vi "RotationApplication v6.vi"() -> ()   [LabVIEW 2012]
uses:
  <instrlib>/ZaberTSeries/Public/Utility/Request.ctl
  <instrlib>/ZaberTSeries/Public/Utility/Response.ctl
  variables/GlobalUI.vi
  <vilib>/Utility/file.llb/Write To Spreadsheet File (string).vi
  Stage Global.vi
  <instrlib>/ZaberTSeries/ZaberTSeries.lvlib
panel:
  in  "OriginalFormula":string
  in  "Restore":bool
  in  "Calibrate":bool
  out "Scanning?":bool
  out "Current Angle (deg)":dbl=45.0
  out "Stage Position (mm)":dbl=76.5
  in  "Time Step (ms)":dbl
  in  "Rotation f(x) (mm -> deg)":string="1*x + -1080.000000"
  in  "Finish Rotation f(x)":bool
  in  "Scan":bool
  in  "stop":bool
  in  "Go Home":bool
  in  "Set Home Offset":dbl=80.0
  in  "TabControl":T1(tab)
  in  "Optimize":bool
  in  "Angle?":bool
  out "Current Angle (deg)":dbl=52.314375
  in  "Move Rel?":bool
  in  "Move Abs?":bool
  in  "Move Rel (deg)":dbl=-1.0 step=0.1
  in  "Move Abs (deg)":dbl=35.0
  in  "Send":bool
  out "Command?":bool=TRUE
  in  "REQUEST:":T2={"Device Number"=1, "Command"=23, "Data"=-10000, "Response Count"=1} {"Command" items=["Echo"=55, "Home"=1, "Move Absolute"=20, "Move Relative"=21, "Move at Constant Speed"=22, "Renumber"=2, "Restore Settings"=36, "Stop"=23]}
  out "Response Data:":T3 {"Command" items=["Constant Speed Tracking"=8, "Echo"=55, "Error"=255, "Home"=1, "Limit Active"=9, "Manual Move Tracking"=10, "Move Absolute"=20, "Move at Constant Speed"=22, "Move Relative"=21, "Renumber"=2, "Restore Settings"=36, "Stop"=23]}
  in  "Command":bool
  in  "DONE":bool
  in  "angle":dbl=7.89375
  in  "Aquire AngleScan":bool
  out "Intensity vs Angle Plot":cluster{dbl[], dbl[]}(graph)={[0.1003125, 0.200625, 0.30093749999999997, 0.40125, 0.5015625, 0.6018749999999999, 0.7021875, 0.8025, 0.9028125, 1.003125, 1.1034374999999998, 1.2037499999999999, 1.3040625, 1.404375, 1.5046875, 1.605, 1.7053125, 1.805625, 1.9059374999999998, 2.00625, 2.1065625, 2.2068749999999997, 2.3071875, 2.4074999999999998, 2.5078125, 2.608125, 2.7084375, 2.80875, 2.9090625, 3.009375, 3.1096874999999997, 3.21, 3.3103124999999998, 3.410625, 3.5109375, 3.61125, 3.7115625, 3.8118749999999997, 3.9121875, 4.0125, 4.1128124999999995, 4.213125, 4.3134375, 4.413749999999999], [0.10330483041158461, 0.10354301638719464, 0.10354301638719464, 0.10358827172256029, 0.10358827172256029, 0.10288562309451152, 0.10288562309451152, 0.10288562309451152, 0.1017709127286577, 0.1017709127286577, 0.10044183498475528, 0.09877691501524301, 0.09877691501524301, 0.10001548208841382, 0.10001548208841382, 0.09941763528963352, 0.09941763528963352, 0.09897222751524294, 0.09965820312499914, 0.09965820312499914, 0.09993807164634047, 0.09985708841463325, 0.09985708841463325, 0.09985708841463325, 0.10042158917682856, 0.10075624047256009, 0.10075624047256009, 0.10102419969512122, 0.1007193216463409, 0.1007193216463409, 0.1007193216463409, 0.10111828315548696, 0.10111828315548696, 0.10111828315548696, 0.10066811166158449, 0.10066811166158449, 0.10040610708841394, 0.10110399199695043, 0.10110399199695043, 0.10115996570121859, 0.10115996570121859, 0.10151248094512112, 0.10151248094512112, 0.10125047637195043]}
  in  "Step Size (deg)":dbl=1.0
  in  "Final Angle (deg)":dbl=45.0
  in  "Initial Angle (deg)":dbl
  in  "Activate AngleScan":bool
  out "Calibrate?":bool
  in  "ABORT":bool
  out "File Destination":path
  in  "Initialize AngleScan":bool
  in  "Simulation":bool
  out "Simulate?":bool
  in  "Finish Stage":bool
  in  "Start/pause":bool
  in  "Start/Pause Stage":bool
  out "Current Position (mm)":dbl
  in  "Finish Rotation":bool
  out "Current Angle":dbl
  in  "Initial Position (mm)":dbl
  in  "Final Position (mm)":dbl
  in  "Number of Steps":u32
  in  "Speed (um/s)":dbl
  in  "Final Angle (deg)":dbl=45.0
  in  "Number of Rotations":u32=4500
  in  "Polynomial Degree":dbl=1.0
  in  "VISA reference name:":refnum<visa-resource-name>="COM4"
  # "==>"
  # "Device"
  # "Command (Binary)"
  # "Data"
  # "==>"
  # "Data"
  # "==>"
  # "Rotation Mount Settings:"
  # "Simulated Delay Stage Settings:"
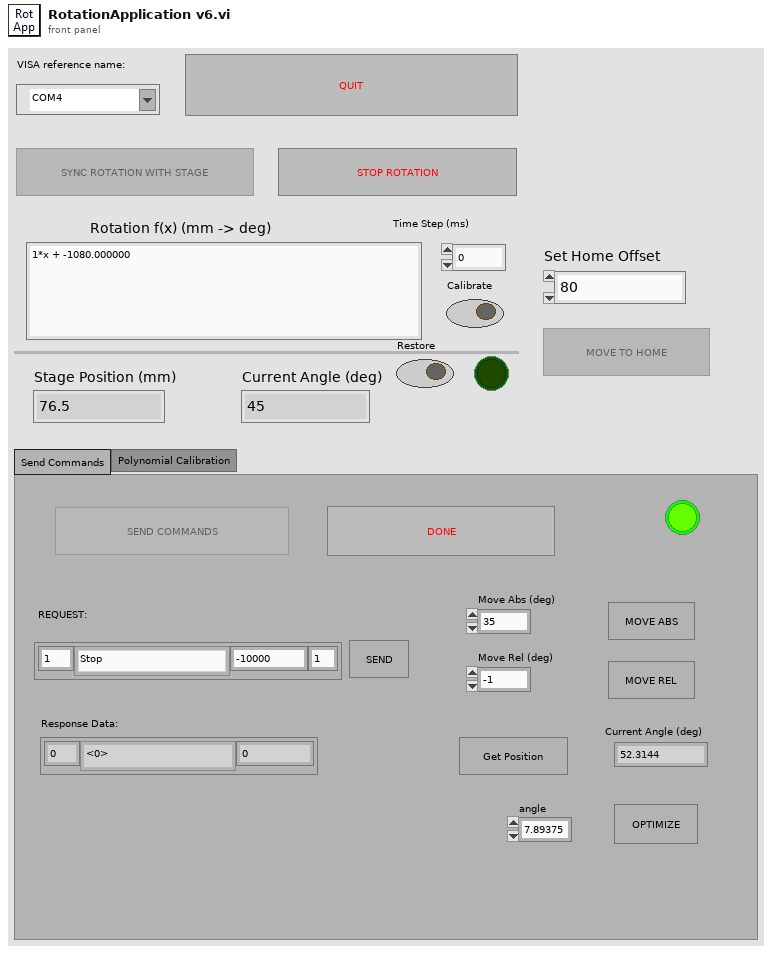
[diagram p1: front panel]
types:
  T1 = enum32{"Send Commands", "Polynomial Calibration", "Simulated f(x)  ", "Adjust Simulation Settings"}
  T2 = typedef "ZaberTSeries.lvlib/Request.ctl" = cluster{"Device Number":u8, "Command":u8, "Data":i32, "Response Count":i32}
  T3 = typedef "ZaberTSeries.lvlib/Response.ctl" = cluster{"Device Number":u8, "Command":u8, "Data":i32}
  T4 = enum8{"Enabled", "Disabled", "Disabled and Grayed Out"}
  T5 = typedef "Scan Parameters.ctl" = cluster{"x pixels":i32, "x voltage min":dbl, "x voltage max":dbl, "y voltage min":dbl, "y voltage max":dbl, "fill frac":dbl, "Zoom":dbl, "BiDi":bool, "scan rate (ms/line)":dbl}
  T6 = typedef "Stage Parameters.ctl" = cluster{"Scan Mode":T7, "Start position mm":dbl, "End position mm":dbl, "Velocity um/sec (continuous)":dbl, "Step size microns (discrete)":dbl, "Frames to grab (grab)":i32, "Sync Rotation with Stage":bool}
  T7 = typedef "ScanMode.ctl" = enum16{"None", "Continuous", "Point Scan (CH3 cursor)", "Point Scan Move (CH3 cursor)", "Grab", "Grab Move Stage", "Grab Move Z-stage", "Cont. Move Z-stage", "Spec Move Stage", "Spec Move Cont", "Surf Calib"}
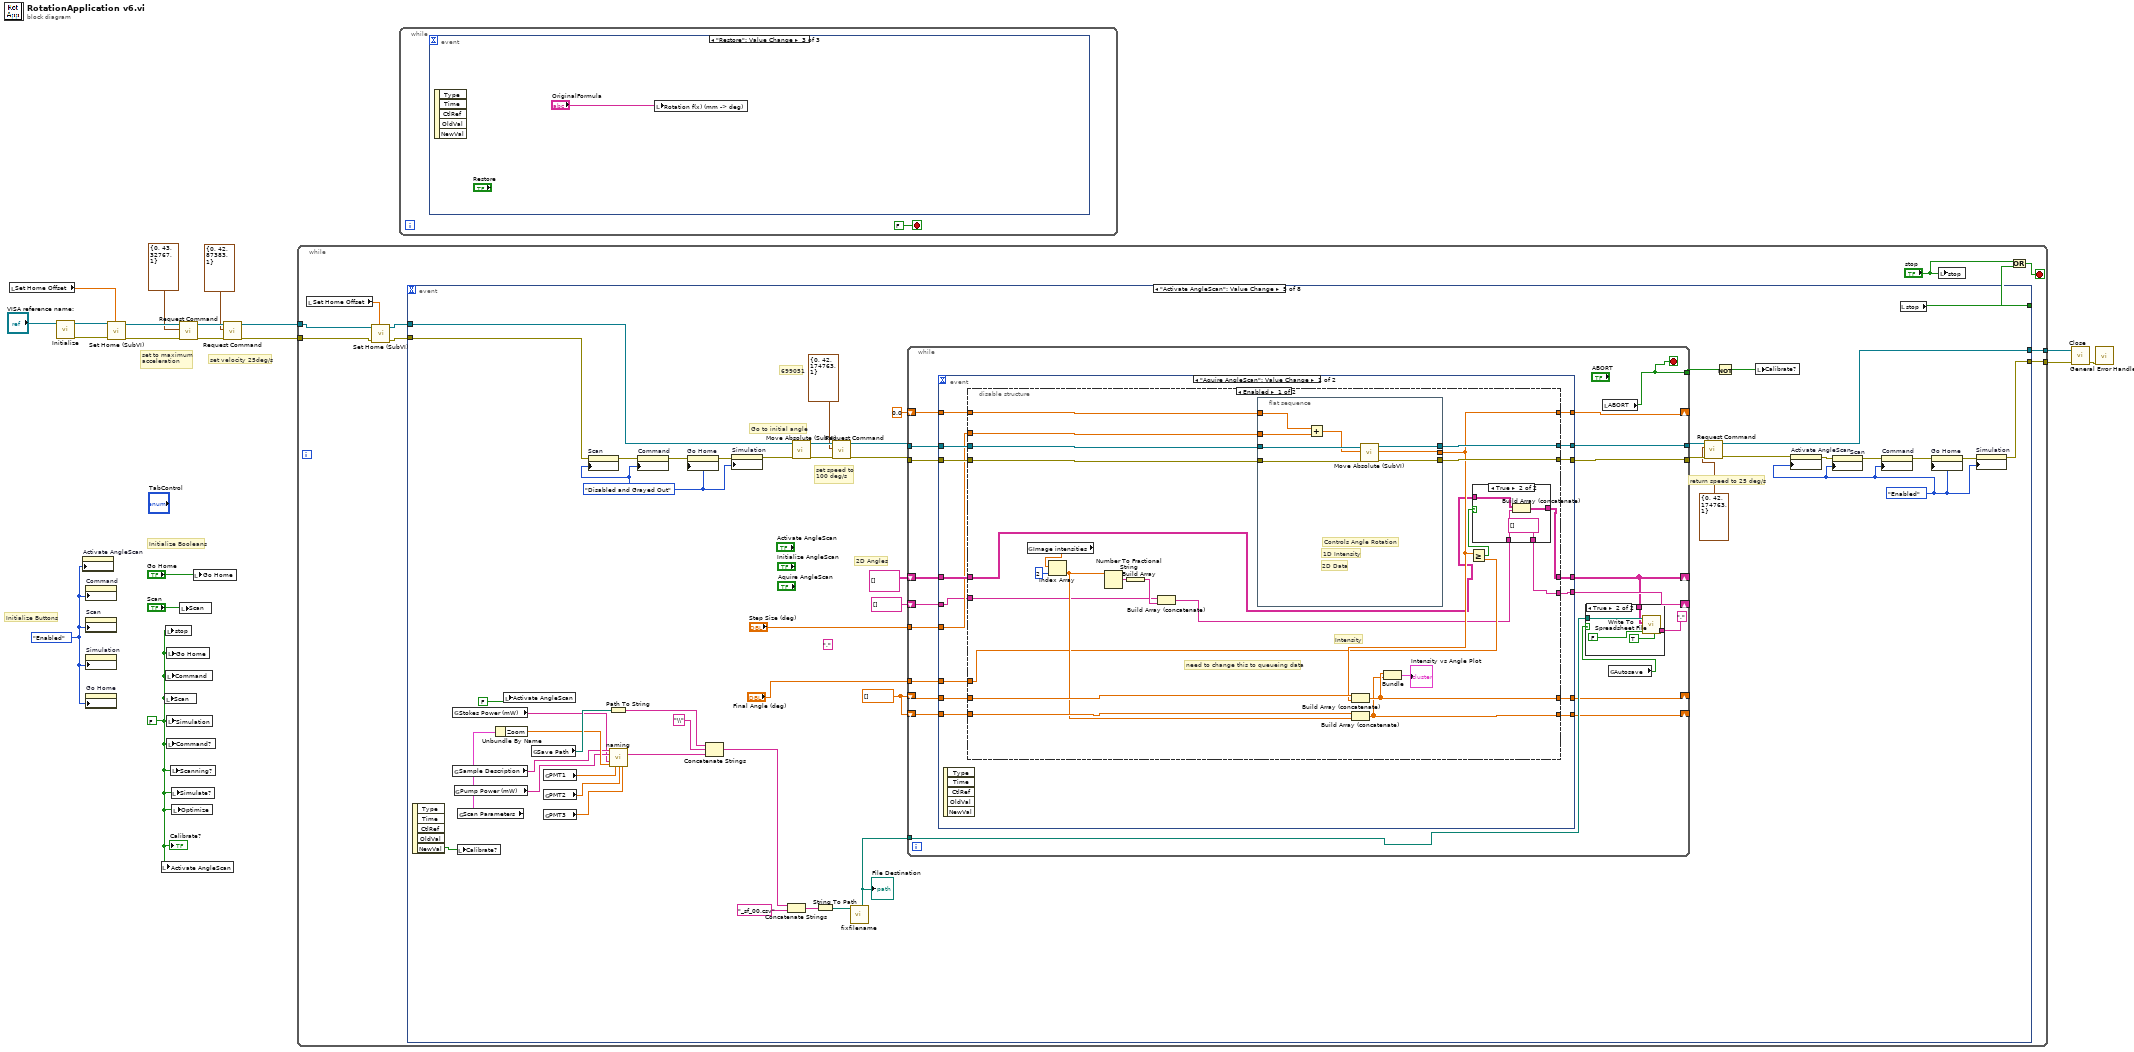
[diagram p0: block diagram]
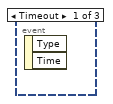
[diagram p2: hidden frame]
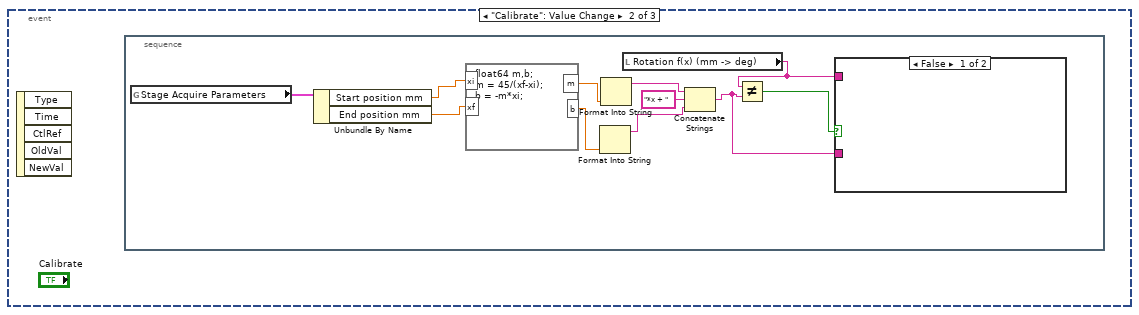
[diagram p3: hidden frame]
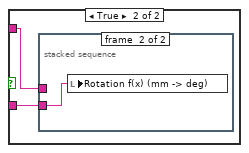
[diagram p4: hidden frame]
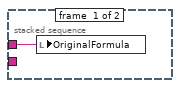
[diagram p5: hidden frame]
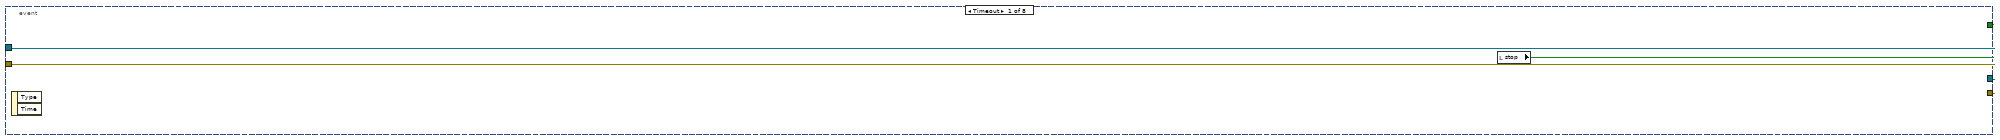
[diagram p6: hidden frame]
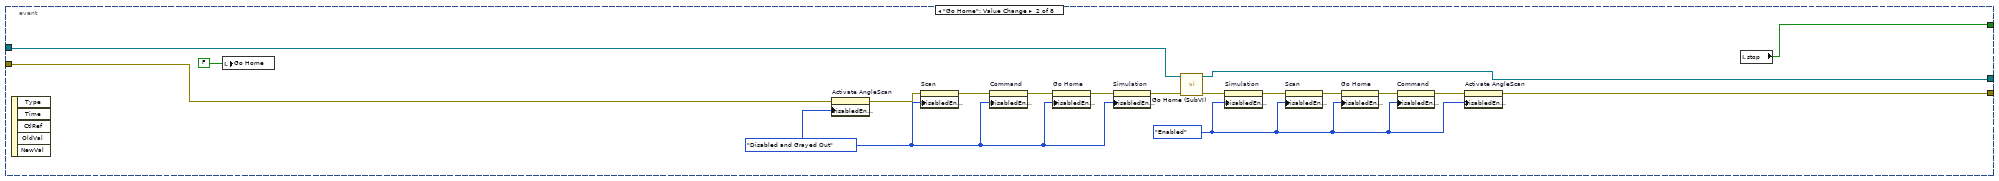
[diagram p7: hidden frame]
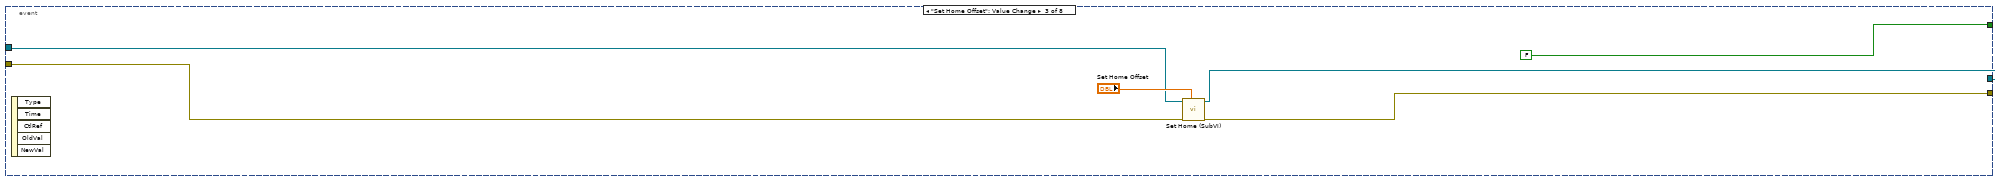
[diagram p8: hidden frame]
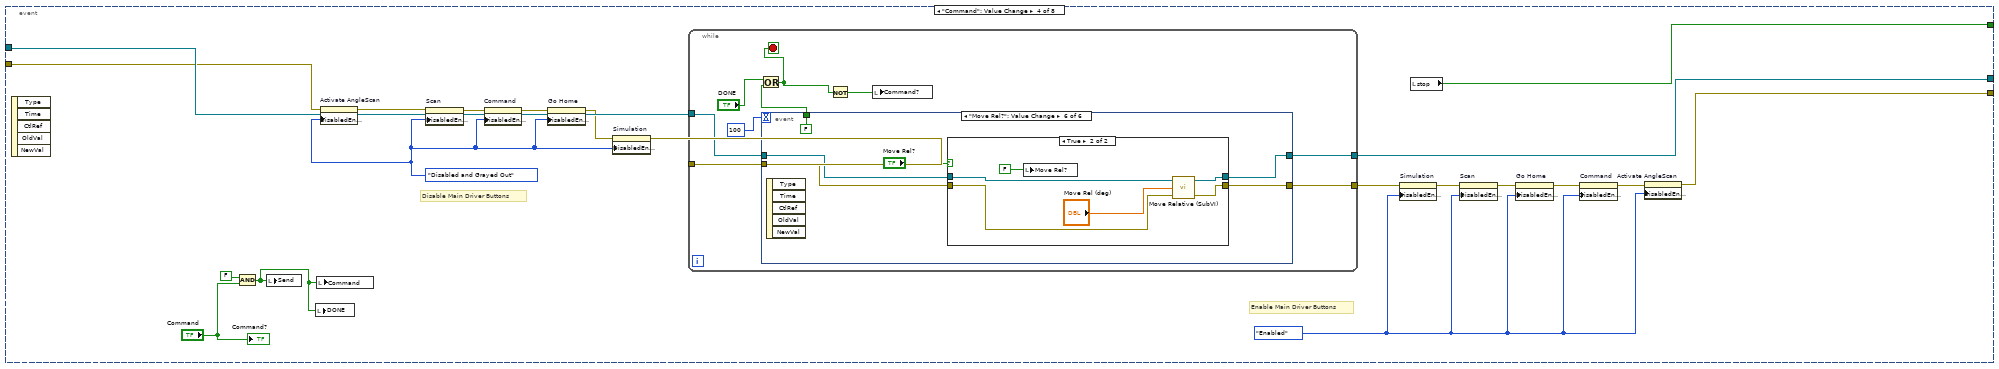
[diagram p9: hidden frame]
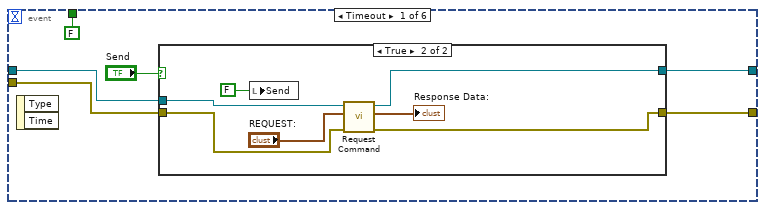
[diagram p10: hidden frame]
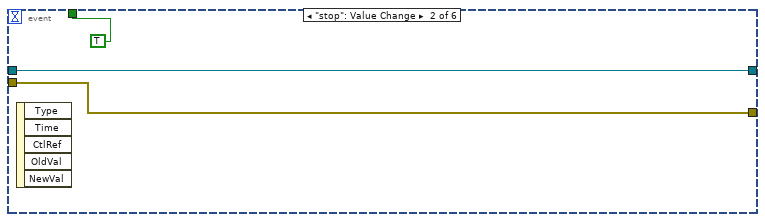
[diagram p12: hidden frame]
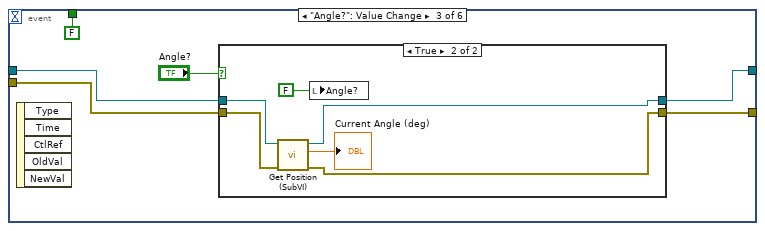
[diagram p13: hidden frame]
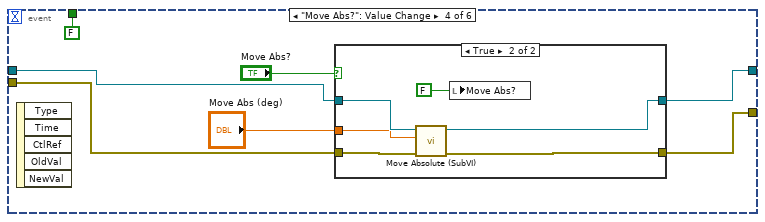
[diagram p15: hidden frame]
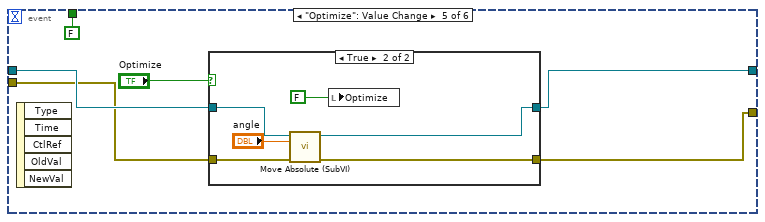
[diagram p17: hidden frame]
diagram:
  w9 = T4."Enabled" ("Disabled")
  w10 = FALSE ("y")
  # "set to maximum\nacceleration"
  # "set velocity 25deg/s"
  # "Initialize Buttons"
  # "Initialize Booleans"
  n1 = local read "Set Home Offset"() -> (w11:dbl)
  n2 = call <instrlib>:"Initialize.vi"("VISA resource name"="VISA reference name:") -> ("error out"=w12:errorcluster, "VISA resource name out"=w13:refnum<visa-resource-name>)  [unwired: 8 in, 1 out]
  n3 = property on="Activate AngleScan" class="Bool (strict)"("DisabledEnum"=w9) -> ()  [unwired: 2 in, 2 out]
  n4 = property on="Command" class="Bool (strict)"("DisabledEnum"=w9) -> ()  [unwired: 2 in, 2 out]
  n5 = property on="Scan" class="Bool (strict)"("DisabledEnum"=w9) -> ()  [unwired: 2 in, 2 out]
  n6 = property on="Simulation" class="Bool (strict)"("DisabledEnum"=w9) -> ()  [unwired: 2 in, 2 out]
  n7 = property on="Go Home" class="Bool (strict)"("DisabledEnum"=w9) -> ()  [unwired: 2 in, 2 out]
  n8 = call "Set Home (SubVI).vi"("Home Offset (deg)"=w11, "error in (no error)"=w12, "VISA Refnum in"=w13) -> ("error out"=w7:errorcluster, "VISA Refnum out"=w8:refnum<visa-resource-name>)  [unwired: 7 in]
  n9 = local write "Activate AngleScan"(w10) -> ()
  n10 = local write "Scan"(w10) -> ()
  n11 = local write "stop"(w10) -> ()
  n12 = local write "Command"(w10) -> ()
  n13 = local write "Go Home"(w10) -> ()
  n14 = local write "Simulation"(w10) -> ()
  n15 = local write "Command?"(w10) -> ()
  n16 = local write "Scanning?"(w10) -> ()
  n17 = local write "Simulate?"(w10) -> ()
  n18 = local write "Optimize"(w10) -> ()
  n19 = call <instrlib>:"Request Command.vi"("error in (no error)"=w7, "Request"=T2 {"Device Number"=0, "Command"=43, "Data"=32767, "Response Count"=1}, "VISA resource name"=w8) -> ("error out"=w5:errorcluster, "VISA resource name out"=w6:refnum<visa-resource-name>)  [unwired: 5 in, 2 out]
  n20 = local write "Scan"("Scan") -> ()
  n21 = local write "Go Home"("Go Home") -> ()
  n22 = call <instrlib>:"Request Command.vi"("error in (no error)"=w5, "Request"=T2 {"Device Number"=0, "Command"=42, "Data"=87383, "Response Count"=1}, "VISA resource name"=w6) -> ("error out"=w3:errorcluster, "VISA resource name out"=w4:refnum<visa-resource-name>)  [unwired: 5 in, 2 out]
  n23 = while {
    tunnel: w4 -> [w23]
    tunnel: w3 -> [w20]
    tunnel: [w29] -> w17
    tunnel: [w28] -> w19
    stop <- w27 stop-if-true
    n24 = local read "Set Home Offset"() -> (w24:dbl)
    n25 = call "Set Home (SubVI).vi"("Home Offset (deg)"=w24, "error in (no error)"=w20, "VISA Refnum in"=w23) -> ("error out"=w21:errorcluster, "VISA Refnum out"=w22:refnum<visa-resource-name>)  [unwired: 7 in]
    n26 = event shown="[4] \"Activate AngleScan\": Value Change" {
      selector: _ -> [_ _ _ _ _ _ _ _]
      dyn-events: _ -> [_ _ _ _ _ _ _ _]
      timeout: _ -> [_ _ _ _ _ _ _ _]
      tunnel: w22 -> [w32 w45 w55 w76 w201 w389 w419 w486]
      tunnel: w21 -> [w31 w36 w54 w62 w205 w386 w404 w485]
      tunnel: [w32 w40 w53 w68 w169 w388 w426 w486] -> w28
      tunnel: [w31 w33 w52 w57 w189 w370 w423 w485] -> w29
      tunnel: [w30 w50 FALSE ("stop") w75 w211 w390 w430 w487] -> w26
      event Timeout {
        n27 = event-data() -> ()  [unwired: 1 in, 2 out]
        n28 = local read "stop"() -> (w30:bool)
      }
      event "Go Home": Value Change {
        w34 = T4."Enabled" ("Disabled")
        w38 = T4."Disabled and Grayed Out" ("Disabled")
        n29 = event-data() -> ()  [unwired: 1 in, 5 out]
        n30 = local write "Go Home"(FALSE ("Go Home")) -> ()
        n31 = property on="Activate AngleScan" class="Bool (strict)"(error in=w36, "DisabledEnum"=w38) -> (error out=w37:errorcluster)  [unwired: 1 in, 1 out]
        n32 = property on="Scan" class="Bool (strict)"(error in=w37, "DisabledEnum"=w38) -> (error out=w48:errorcluster)  [unwired: 1 in, 1 out]
        n33 = property on="Command" class="Bool (strict)"(error in=w48, "DisabledEnum"=w38) -> (error out=w47:errorcluster)  [unwired: 1 in, 1 out]
        n34 = property on="Go Home" class="Bool (strict)"(error in=w47, "DisabledEnum"=w38) -> (error out=w46:errorcluster)  [unwired: 1 in, 1 out]
        n35 = property on="Simulation" class="Bool (strict)"(error in=w46, "DisabledEnum"=w38) -> (error out=w44:errorcluster)  [unwired: 1 in, 1 out]
        n36 = call "Go Home (SubVI).vi"("error in (no error)"=w44, "VISA Refnum in"=w45) -> ("error out"=w39:errorcluster, "VISA Refnum out"=w40:refnum<visa-resource-name>)  [unwired: 8 in]
        n37 = property on="Simulation" class="Bool (strict)"(error in=w39, "DisabledEnum"=w34) -> (error out=w41:errorcluster)  [unwired: 1 in, 1 out]
        n38 = property on="Scan" class="Bool (strict)"(error in=w41, "DisabledEnum"=w34) -> (error out=w43:errorcluster)  [unwired: 1 in, 1 out]
        n39 = property on="Go Home" class="Bool (strict)"(error in=w43, "DisabledEnum"=w34) -> (error out=w42:errorcluster)  [unwired: 1 in, 1 out]
        n40 = property on="Command" class="Bool (strict)"(error in=w42, "DisabledEnum"=w34) -> (error out=w35:errorcluster)  [unwired: 1 in, 1 out]
        n41 = property on="Activate AngleScan" class="Bool (strict)"(error in=w35, "DisabledEnum"=w34) -> (error out=w33:errorcluster)  [unwired: 1 in, 1 out]
        n42 = local read "stop"() -> (w50:bool)
      }
      event "Set Home Offset": Value Change {
        n43 = event-data() -> ()  [unwired: 1 in, 5 out]
        n44 = call "Set Home (SubVI).vi"("Home Offset (deg)"="Set Home Offset", "error in (no error)"=w54, "VISA Refnum in"=w55) -> ("error out"=w52:errorcluster, "VISA Refnum out"=w53:refnum<visa-resource-name>)  [unwired: 7 in]
      }
      event "Command": Value Change {
        w59 = T4."Enabled" ("Disabled")
        w60 = T4."Disabled and Grayed Out" ("Disabled")
        # "Enable Main Driver Buttons"
        # "Disable Main Driver Buttons"
        n45 = event-data() -> ()  [unwired: 1 in, 5 out]
        n46 = And(x=FALSE ("Command"), y="Command") -> (x .and. y?=w64:bool)
        n47 = local write "Send"(w64) -> ()
        n48 = local write "DONE"(w64) -> ()
        n49 = local write "Command"(w64) -> ()
        n50 = property on="Activate AngleScan" class="Bool (strict)"(error in=w62, "DisabledEnum"=w60) -> (error out=w61:errorcluster)  [unwired: 1 in, 1 out]
        n51 = property on="Scan" class="Bool (strict)"(error in=w61, "DisabledEnum"=w60) -> (error out=w70:errorcluster)  [unwired: 1 in, 1 out]
        n52 = property on="Command" class="Bool (strict)"(error in=w70, "DisabledEnum"=w60) -> (error out=w71:errorcluster)  [unwired: 1 in, 1 out]
        n53 = property on="Go Home" class="Bool (strict)"(error in=w71, "DisabledEnum"=w60) -> (error out=w72:errorcluster)  [unwired: 1 in, 1 out]
        n54 = property on="Simulation" class="Bool (strict)"(error in=w72, "DisabledEnum"=w60) -> (error out=w69:errorcluster)  [unwired: 1 in, 1 out]
        n55 = while {
          tunnel: w76 -> [w82]
          tunnel: [w85] -> w68
          tunnel: w69 -> [w81]
          tunnel: [w84] -> w63
          stop <- w78 stop-if-true
          n56 = event shown="[5] \"Move Rel?\": Value Change" {
            selector: _ -> [_ _ _ _ _ _]
            dyn-events: _ -> [_ _ _ _ _ _]
            timeout: 100 -> [_ _ _ _ _ _]
            tunnel: [w91 w102 w108 w121 w135 w149] -> w85
            tunnel: [w90 w103 w105 w119 w134 w148] -> w84
            tunnel: w82 -> [w88 w102 w107 w122 w137 w151]
            tunnel: w81 -> [w87 w103 w106 w120 w136 w150]
            tunnel: [FALSE TRUE FALSE FALSE FALSE FALSE] -> w77
            event Timeout {
              n57 = event-data() -> ()  [unwired: 1 in, 2 out]
              n58 = case shown="True" "Send" {
                tunnel: w88 -> [w93 w99]
                tunnel: [w93 w98] -> w91
                tunnel: w87 -> [w92 w97]
                tunnel: [w92 w96] -> w90
                frame False {
                }
                frame True {
                  n59 = local write "Send"(FALSE ("Send")) -> ()
                  n60 = call <instrlib>:"Request Command.vi"("error in (no error)"=w97, "Request"="REQUEST:", "VISA resource name"=w99) -> ("error out"=w96:errorcluster, "First Response"=→"Response Data:":T3, "VISA resource name out"=w98:refnum<visa-resource-name>)  [unwired: 5 in, 1 out]
                }
              }
            }
            event "stop": Value Change {
              n61 = event-data() -> ()  [unwired: 1 in, 5 out]
            }
            event "Angle?": Value Change {
              n62 = event-data() -> ()  [unwired: 1 in, 5 out]
              n63 = case shown="True" "Angle?" {
                tunnel: [w111 w116] -> w108
                tunnel: w107 -> [w111 w115]
                tunnel: w106 -> [w110 w114]
                tunnel: [w110 w113] -> w105
                frame False {
                }
                frame True {
                  n64 = call "Get Position (SubVI).vi"("error in (no error)"=w114, "VISA Refnum in"=w115) -> ("error out"=w113:errorcluster, "Position"=→"Current Angle (deg)":dbl, "VISA Refnum out"=w116:refnum<visa-resource-name>)  [unwired: 7 in]
                  n65 = local write "Angle?"(FALSE ("Angle?")) -> ()
                }
              }
            }
            event "Move Abs?": Value Change {
              n66 = event-data() -> ()  [unwired: 1 in, 5 out]
              n67 = case shown="True" "Move Abs?" {
                tunnel: "Move Abs (deg)" -> [_ w128]
                tunnel: w122 -> [w126 w132]
                tunnel: [w126 w131] -> w121
                tunnel: w120 -> [w125 w130]
                tunnel: [w125 w129] -> w119
                frame False {
                }
                frame True {
                  n68 = call "Move Absolute (SubVI).vi"("error in (no error)"=w130, "Move to Angle"=w128, "VISA Refnum in"=w132) -> ("error out"=w129:errorcluster, "VISA Refnum out"=w131:refnum<visa-resource-name>)  [unwired: 6 in, 1 out]
                  n69 = local write "Move Abs?"(FALSE ("Move Abs?")) -> ()
                }
              }
            }
            event "Optimize": Value Change {
              n70 = event-data() -> ()  [unwired: 1 in, 5 out]
              n71 = case shown="True" "Optimize" {
                tunnel: w137 -> [w140 w146]
                tunnel: [w140 w145] -> w135
                tunnel: w136 -> [w139 w144]
                tunnel: [w139 w143] -> w134
                frame False {
                }
                frame True {
                  n72 = call "Move Absolute (SubVI).vi"("error in (no error)"=w144, "Move to Angle"="angle", "VISA Refnum in"=w146) -> ("error out"=w143:errorcluster, "VISA Refnum out"=w145:refnum<visa-resource-name>)  [unwired: 6 in, 1 out]
                  n73 = local write "Optimize"(FALSE ("Move Abs?")) -> ()
                }
              }
            }
            event "Move Rel?": Value Change {
              n74 = event-data() -> ()  [unwired: 1 in, 5 out]
              n75 = case shown="True" "Move Rel?" {
                tunnel: w151 -> [w154 w159]
                tunnel: w150 -> [w153 w158]
                tunnel: [w154 w156] -> w149
                tunnel: [w153 w157] -> w148
                frame False {
                }
                frame True {
                  n76 = local write "Move Rel?"(FALSE ("Move Rel?")) -> ()
                  n77 = call "Move Relative (SubVI).vi"("error in (no error)"=w158, "Degrees to move"="Move Rel (deg)", "VISA resource name"=w159) -> ("error out"=w157:errorcluster, "VISA resource name out"=w156:refnum<visa-resource-name>)  [unwired: 1 out]
                }
              }
            }
          }
          n78 = Or(x="DONE", y=w77) -> (x .or. y?=w78:bool)
          n79 = Not(x=w78) -> (.not. x?=w83:bool)
          n80 = local write "Command?"(w83) -> ()
        }
        n81 = property on="Simulation" class="Bool (strict)"(error in=w63, "DisabledEnum"=w59) -> (error out=w65:errorcluster)  [unwired: 1 in, 1 out]
        n82 = local read "stop"() -> (w75:bool)
        n83 = property on="Scan" class="Bool (strict)"(error in=w65, "DisabledEnum"=w59) -> (error out=w67:errorcluster)  [unwired: 1 in, 1 out]
        n84 = property on="Go Home" class="Bool (strict)"(error in=w67, "DisabledEnum"=w59) -> (error out=w66:errorcluster)  [unwired: 1 in, 1 out]
        n85 = property on="Command" class="Bool (strict)"(error in=w66, "DisabledEnum"=w59) -> (error out=w58:errorcluster)  [unwired: 1 in, 1 out]
        n86 = property on="Activate AngleScan" class="Bool (strict)"(error in=w58, "DisabledEnum"=w59) -> (error out=w57:errorcluster)  [unwired: 1 in, 1 out]
        "Command?" <- "Command"
      }
      event "Activate AngleScan": Value Change {
        w171 = dbl[] []
        (unwired) "," ("delimiter (\\t)")
        w198 = T4."Enabled" ("Disabled")
        w199 = T4."Disabled and Grayed Out" ("Disabled")
        # "return speed to 25 deg/s"
        # "699051"
        # "set speed to\n100 deg/s"
        # "2D Angles"
        # "Go to initial angle"
        n87 = event-data() -> ("NewVal"=w210:bool)  [unwired: 1 in, 4 out]
        n88 = global read "GlobalUI.vi" "Stokes Power (mW)"() -> (w174:string)
        n89 = global read "GlobalUI.vi" "Sample Description"() -> (w176:string)
        n90 = global read "GlobalUI.vi" "Pump Power (mW)"() -> (w175:string)
        n91 = local write "Calibrate?"(w210) -> ()
        n92 = global read "GlobalUI.vi" "Scan Parameters"() -> (w178:T5)
        n93 = Unbundle By Name(w178) -> ("Zoom"=w177:dbl)
        n94 = local write "Activate AngleScan"(FALSE ("Scan Angles")) -> ()
        n95 = global read "GlobalUI.vi" "Save Path"() -> (w182:path)
        n96 = global read "GlobalUI.vi" "PMT1"() -> (w181:dbl)
        n97 = global read "GlobalUI.vi" "PMT2"() -> (w180:dbl)
        n98 = global read "GlobalUI.vi" "PMT3"() -> (w179:dbl)
        n99 = property on="Scan" class="Bool (strict)"(error in=w205, "DisabledEnum"=w199) -> (error out=w207:errorcluster)  [unwired: 1 in, 1 out]
        n100 = Path To String(path=w182) -> (string=w187:string)
        n101 = call "naming.vi"("Sample Description"=w176, "Pump Power (mW)"=w175, "Stokes Power (mW)"=w174, "Zoom"=w177, "PMT1"=w181, "PMT2"=w180, "PMT3"=w179) -> ("filename"=w173:string)  [unwired: 8 in]
        n102 = property on="Command" class="Bool (strict)"(error in=w207, "DisabledEnum"=w199) -> (error out=w208:errorcluster)  [unwired: 1 in, 1 out]
        n103 = property on="Go Home" class="Bool (strict)"(error in=w208, "DisabledEnum"=w199) -> (error out=w206:errorcluster)  [unwired: 1 in, 1 out]
        n104 = Concatenate Strings(w187, "\\" ("string"), w173) -> (w183:string)
        n105 = property on="Simulation" class="Bool (strict)"(error in=w206, "DisabledEnum"=w199) -> (error out=w200:errorcluster)  [unwired: 1 in, 1 out]
        n106 = Concatenate Strings(w183, "_sf_00.csv" ("string")) -> (w185:string)
        n107 = call "Move Absolute (SubVI).vi"("error in (no error)"=w200, "VISA Refnum in"=w201) -> ("error out"=w191:errorcluster, "VISA Refnum out"=w194:refnum<visa-resource-name>)  [unwired: 7 in, 1 out]
        n108 = String To Path(string=w185) -> (path=w184:path)
        n109 = call <instrlib>:"Request Command.vi"("error in (no error)"=w191, "Request"=T2 {"Device Number"=0, "Command"=42, "Data"=174763, "Response Count"=1}, "VISA resource name"=w194) -> ("error out"=w192:errorcluster, "VISA resource name out"=w193:refnum<visa-resource-name>)  [unwired: 5 in, 2 out]
        n110 = call "fixfilename.vi"("Path"=w184) -> ("fixed path"=w172:path)  [unwired: 9 in, 1 out]
        "File Destination" <- w172
        n111 = while {
          tunnel: "Final Angle (deg)" -> [w230]
          tunnel: w192 -> [w231]
          tunnel: [w217] -> w168
          tunnel: [w218] -> w170
          shift-right: [w213] -> _
          shift-left: string[][] [] -> [w229]
          tunnel: [w225] -> w197
          tunnel: w193 -> [w228]
          tunnel: w172 -> [w226]
          shift-right: [w224] -> _
          shift-left: 0.0 ("Initial Angle (deg)") -> [w223]
          shift-right: [w220] -> _
          shift-left: w171 -> [w222]
          shift-right: [w219] -> _
          shift-left: w171 -> [w221]
          tunnel: "Step Size (deg)" -> [w216]
          shift-right: [w215] -> _
          shift-left: string[] [] -> [w214]
          stop <- w225 stop-if-true
          n112 = event shown="[0] \"Aquire AngleScan\": Value Change" {
            selector: _ -> [_ _]
            dyn-events: _ -> [_ _]
            timeout: _ -> [_ _]
            tunnel: w228 -> [w252 _]
            tunnel: w231 -> [w251 _]
            tunnel: [w250 _] -> w218
            tunnel: [w249 _] -> w217
            tunnel: w230 -> [w248 w358]
            tunnel: w223 -> [w246 _]
            tunnel: w229 -> [w247 _]
            tunnel: [w245 w350] -> w213
            tunnel: [w244 "Initial Angle (deg)"] -> w224
            tunnel: w222 -> [w243 _]
            tunnel: w221 -> [w242 _]
            tunnel: [w241 _] -> w220
            tunnel: [w240 _] -> w219
            tunnel: w216 -> [w239 w354]
            tunnel: [w237 w351] -> w215
            tunnel: w214 -> [w238 _]
            event "Aquire AngleScan": Value Change {
              n113 = event-data() -> ()  [unwired: 1 in, 5 out]
              n114 = disable-structure shown="Enabled" {
                disable-tunnel: w239 -> [w261 w313]
                disable-tunnel: w252 -> [w276 w312]
                disable-tunnel: w251 -> [w275 w311]
                disable-tunnel: [w274 w310] -> w250
                disable-tunnel: [w273 w309] -> w249
                disable-tunnel: w248 -> [w258 w308]
                disable-tunnel: w247 -> [w256 w307]
                disable-tunnel: w246 -> [w272 w298]
                disable-tunnel: [w254 w296] -> w245
                disable-tunnel: [w259 w294] -> w244
                disable-tunnel: w243 -> [w271 _]
                disable-tunnel: w242 -> [w270 _]
                disable-tunnel: [w269 w293] -> w241
                disable-tunnel: [w268 w292] -> w240
                disable-tunnel: w238 -> [w260 _]
                disable-tunnel: [w253 _] -> w237
                frame Enabled {
                  # "need to change this to queueing data"
                  # "Intensity"
                  n115 = global read "GlobalUI.vi" "Image intensities"() -> (w267:dbl[])
                  n116 = Index Array(array=w267, index=2) -> (element=w265:dbl)
                  n117 = Number To Fractional String(number=w265) -> (F-format string=w263:string)  [unwired: 3 in]
                  n118 = Build Array(w263) -> (w262:string[])
                  n119 = Build Array (concatenate)(w260, w262) -> (w255:string[])
                  n120 = flat-sequence {
                    tunnel: w276 -> [w290]
                    tunnel: w275 -> [w289]
                    tunnel: [w288] -> w274
                    tunnel: [w287] -> w273
                    tunnel: w272 -> [w284]
                    tunnel: [w285] -> w259
                    tunnel: w261 -> [w283]
                    frame #0 {
                      # "1D Intensity"
                      # "2D Data"
                      # "Controls Angle Rotation"
                      n121 = Add(x=w284, y=w283) -> (x+y=w286:dbl)
                      n122 = call "Move Absolute (SubVI).vi"("error in (no error)"=w289, "Move to Angle"=w286, "VISA Refnum in"=w290) -> ("error out"=w287:errorcluster, "New Angle"=w285:dbl, "VISA Refnum out"=w288:refnum<visa-resource-name>)  [unwired: 6 in]
                    }
                  }
                  n123 = Build Array (concatenate)(w270, w265) -> (w268:dbl[])
                  n124 = Build Array (concatenate)(w271, w259) -> (w269:dbl[])
                  n125 = Bundle(w269, w268) -> (→"Intensity vs Angle Plot":cluster{dbl[], dbl[]})  [unwired: 1 in]
                  n126 = Greater Or Equal?(x=w259, y=w258) -> (x >= y?=w257:bool)
                  n127 = case shown="True" w257 {
                    tunnel: w256 -> [w278 w282]
                    tunnel: w255 -> [w277 w281]
                    tunnel: [w278 w280] -> w254
                    tunnel: [w277 string[] []] -> w253
                    frame False {
                    }
                    frame True {
                      n128 = Build Array (concatenate)(w282, w281) -> (w280:string[][])
                    }
                  }
                }
                frame Disabled {
                  w291 = dbl[] []
                  n129 = global read "GlobalUI.vi" "Stage Position (mm)"() -> (w302:dbl)
                  n130 = global read "GlobalUI.vi" "Image intensities"() -> (w306:dbl[])
                  n131 = Index Array(array=w306, index=2) -> (element=w304:dbl)
                  n132 = Number To Fractional String(number=w302) -> (F-format string=w301:string)  [unwired: 3 in]
                  n133 = Number To Fractional String(number=w304) -> (F-format string=w295:string)  [unwired: 3 in]
                  n134 = Build Array(w301) -> (w300:string[])
                  n135 = Build Array (concatenate)(w300, w295) -> (w299:string[])
                  n136 = while {
                    tunnel: w313 -> [w339]
                    tunnel: w312 -> [w338]
                    tunnel: w311 -> [w337]
                    tunnel: [w336] -> w310
                    tunnel: [w335] -> w309
                    tunnel: w308 -> [w334]
                    tunnel: w307 -> [w326]
                    shift-right: [w330] -> w303
                    shift-left: w299 -> [w328]
                    shift-right: [w321] -> w292
                    shift-left: w291 -> [w324]
                    shift-right: [w322] -> w293
                    shift-left: w291 -> [w323]
                    shift-right: [w319] -> w294
                    shift-left: w298 -> [w318]
                    tunnel: [w315] -> w297
                    stop <- w317 stop-if-true
                    # "Intensity"
                    n137 = flat-sequence {
                      tunnel: w339 -> [w341]
                      tunnel: w338 -> [w349]
                      tunnel: w337 -> [w348]
                      tunnel: [w347] -> w336
                      tunnel: [w346] -> w335
                      tunnel: w318 -> [w342]
                      tunnel: w328 -> [w344]
                      tunnel: [w344] -> w327
                      tunnel: w326 -> [w340]
                      tunnel: [w343] -> w319
                      tunnel: [w340] -> w315
                      frame #0 {
                        # "1D Intensity"
                        # "2D Data"
                        # "Controls Angle Rotation"
                        n138 = Add(x=w342, y=w341) -> (x+y=w345:dbl)
                        n139 = call "Move Absolute (SubVI).vi"("error in (no error)"=w348, "Move to Angle"=w345, "VISA Refnum in"=w349) -> ("error out"=w346:errorcluster, "New Angle"=w343:dbl, "VISA Refnum out"=w347:refnum<visa-resource-name>)  [unwired: 6 in]
                      }
                    }
                    n140 = Wait (ms)(milliseconds to wait=u32 10) -> ()  [unwired: 1 out]
                    n141 = global read "GlobalUI.vi" "Image intensities"() -> (w332:dbl[])
                    n142 = Index Array(array=w332, index=2) -> (element=w325:dbl)
                    n143 = Build Array (concatenate)(w324, w325) -> (w321:dbl[])
                    n144 = Build Array (concatenate)(w323, w319) -> (w322:dbl[])
                    n145 = local read "ABORT"() -> (w314:bool)
                    n146 = Greater Or Equal?(x=w319, y=w334) -> (x >= y?=w333:bool)
                    n147 = Bundle(w322, w321) -> (w320:cluster{dbl[], dbl[]})  [unwired: 1 in]
                    n148 = Number To Fractional String(number=w325) -> (F-format string=w329:string)  [unwired: 3 in]
                    n149 = Build Array (concatenate)(w327, w329) -> (w330:string[])
                    n150 = Or(x=w333, y=w314) -> (x .or. y?=w317:bool)
                  }
                  n151 = Build Array (concatenate)(w297, w303) -> (w296:string[][])
                }
              }
            }
            event "Initialize AngleScan": Value Change {
              # "Initialize Angle Array"
              n152 = event-data() -> ()  [unwired: 1 in, 5 out]
              n153 = Build Array("theta (deg)") -> (w357:string[])
              n154 = Build Array (concatenate)(w357) -> (w355:string[])
              n155 = while {
                shift-right: [w365] -> _
                shift-left: "Initial Angle (deg)" -> [w361]
                tunnel: w358 -> [w364]
                shift-right: [w367] -> w360
                shift-left: w355 -> [w368]
                tunnel: w354 -> [w363]
                stop <- w369 stop-if-true
                n156 = Add(x=w361, y=w363) -> (x+y=w365:dbl)
                n157 = Add(x=w361, y=w363) -> (x+y=w362:dbl)
                n158 = Number To Fractional String(number=w361) -> (F-format string=w366:string)  [unwired: 3 in]
                n159 = Greater?(x=w362, y=w364) -> (0:w369:bool)
                n160 = Build Array (concatenate)(w368, w366) -> (w367:string[])
              }
              n161 = Build Array(w360) -> (w350:string[][])
              n162 = global read "GlobalUI.vi" "Stage Position (mm)"() -> (w352:dbl)
              n163 = Number To Fractional String(number=w352) -> (F-format string=w353:string)  [unwired: 3 in]
              n164 = Build Array(w353) -> (w351:string[])
            }
          }
          n165 = local read "ABORT"() -> (w225:bool)
          n166 = global read "GlobalUI.vi" "Autosave"() -> (w212:bool)
          n167 = case shown="True" w212 {
            tunnel: "," ("delimiter (\\t)") -> [_ w236]
            tunnel: w226 -> [_ w235]
            tunnel: w213 -> [_ w232]
            frame False {
            }
            frame True {
              n168 = call-poly <vilib>:"Write To Spreadsheet File.vi"("delimiter (\\t)"=w236, "transpose? (no:F)"=TRUE, "append to file? (new file:F)"=FALSE, "2D data"=w232, "file path (dialog if empty)"=w235) -> ()  [unwired: 3 in, 1 out]
            }
          }
        }
        n169 = call <instrlib>:"Request Command.vi"("error in (no error)"=w168, "Request"=T2 {"Device Number"=0, "Command"=42, "Data"=174763, "Response Count"=1}, "VISA resource name"=w170) -> ("error out"=w167:errorcluster, "VISA resource name out"=w169:refnum<visa-resource-name>)  [unwired: 5 in, 2 out]
        n170 = Not(x=w197) -> (.not. x?=w196:bool)
        n171 = local write "Calibrate?"(w196) -> ()
        n172 = property on="Activate AngleScan" class="Bool (strict)"(error in=w167, "DisabledEnum"=w198) -> (error out=w195:errorcluster)  [unwired: 1 in, 1 out]
        n173 = property on="Scan" class="Bool (strict)"(error in=w195, "DisabledEnum"=w198) -> (error out=w203:errorcluster)  [unwired: 1 in, 1 out]
        n174 = property on="Command" class="Bool (strict)"(error in=w203, "DisabledEnum"=w198) -> (error out=w204:errorcluster)  [unwired: 1 in, 1 out]
        n175 = local read "stop"() -> (w211:bool)
        n176 = property on="Go Home" class="Bool (strict)"(error in=w204, "DisabledEnum"=w198) -> (error out=w202:errorcluster)  [unwired: 1 in, 1 out]
        n177 = property on="Simulation" class="Bool (strict)"(error in=w202, "DisabledEnum"=w198) -> (error out=w189:errorcluster)  [unwired: 1 in, 1 out]
      }
      event "Scan": Value Change {
        w371 = T4."Enabled" ("Disabled")
        w373 = T4."Disabled and Grayed Out" ("Disabled")
        n178 = event-data() -> ()  [unwired: 1 in, 5 out]
        n179 = local read "Scan"() -> (→"Scanning?":bool)
        n180 = property on="Scan" class="Bool (strict)"(error in=w386, "DisabledEnum"=w373) -> (error out=w385:errorcluster)  [unwired: 1 in, 1 out]
        n181 = local write "Finish Rotation f(x)"(FALSE ("Command")) -> ()
        n182 = property on="Command" class="Bool (strict)"(error in=w385, "DisabledEnum"=w373) -> (error out=w387:errorcluster)  [unwired: 1 in, 1 out]
        n183 = property on="Go Home" class="Bool (strict)"(error in=w387, "DisabledEnum"=w373) -> (error out=w382:errorcluster)  [unwired: 1 in, 1 out]
        n184 = property on="Simulation" class="Bool (strict)"(error in=w382, "DisabledEnum"=w373) -> (error out=w375:errorcluster)  [unwired: 1 in, 1 out]
        n185 = property on="Activate AngleScan" class="Bool (strict)"(error in=w375, "DisabledEnum"=w373) -> (error out=w374:errorcluster)  [unwired: 1 in, 1 out]
        n186 = while {
          tunnel: w389 -> [w400]
          tunnel: [w399] -> w388
          tunnel: w374 -> [w398]
          tunnel: [w397] -> w380
          tunnel: ["Finish Rotation f(x)"] -> w376
          stop <- "Finish Rotation f(x)" stop-if-true
          n187 = call "Simple Function (SubVI).vi"("f(x) (mm -> deg)"="Rotation f(x) (mm -> deg)") -> ("Stage Position (mm)"=→"Stage Position (mm)":dbl, "Next Angle (deg)"=w394:dbl)  [unwired: 9 in]
          n188 = call "Move Absolute (SubVI).vi"("error in (no error)"=w398, "Move to Angle"=w394, "VISA Refnum in"=w400) -> ("error out"=w397:errorcluster, "New Angle"=→"Current Angle (deg)":dbl, "VISA Refnum out"=w399:refnum<visa-resource-name>)  [unwired: 6 in]
          n189 = Wait (ms)(milliseconds to wait="Time Step (ms)") -> ()  [unwired: 1 out]
        }
        n190 = Not(x=w376) -> (.not. x?=w377:bool)
        n191 = property on="Simulation" class="Bool (strict)"(error in=w380, "DisabledEnum"=w371) -> (error out=w381:errorcluster)  [unwired: 1 in, 1 out]
        n192 = local write "Finish Rotation f(x)"(w377) -> ()
        n193 = local write "Scanning?"(w377) -> ()
        n194 = local write "Scan"(w377) -> ()
        n195 = property on="Scan" class="Bool (strict)"(error in=w381, "DisabledEnum"=w371) -> (error out=w383:errorcluster)  [unwired: 1 in, 1 out]
        n196 = property on="Go Home" class="Bool (strict)"(error in=w383, "DisabledEnum"=w371) -> (error out=w384:errorcluster)  [unwired: 1 in, 1 out]
        n197 = local read "stop"() -> (w390:bool)
        n198 = property on="Command" class="Bool (strict)"(error in=w384, "DisabledEnum"=w371) -> (error out=w372:errorcluster)  [unwired: 1 in, 1 out]
        n199 = property on="Activate AngleScan" class="Bool (strict)"(error in=w372, "DisabledEnum"=w371) -> (error out=w370:errorcluster)  [unwired: 1 in, 1 out]
      }
      event "Simulation": Value Change {
        w413 = -1
        w412 = -1
        w403 = T4."Enabled" ("Disabled")
        w406 = T4."Disabled and Grayed Out" ("Disabled")
        n200 = event-data() -> ()  [unwired: 1 in, 5 out]
        n201 = property on="Activate AngleScan" class="Bool (strict)"(error in=w404, "DisabledEnum"=w406) -> (error out=w405:errorcluster)  [unwired: 1 in, 1 out]
        n202 = And(x=FALSE ("Command"), y="Simulation") -> (x .and. y?=w407:bool)
        n203 = global write "Stage Global.vi" "Position"("Initial Position (mm)") -> ()
        n204 = global write "Stage Global.vi" "Initial Position"("Initial Position (mm)") -> ()
        n205 = local write "Current Position (mm)"("Initial Position (mm)") -> ()
        n206 = local write "Simulation"(w407) -> ()
        n207 = local write "Start/pause"(w407) -> ()
        n208 = local write "Start/Pause Stage"(w407) -> ()
        n209 = property on="Scan" class="Bool (strict)"(error in=w405, "DisabledEnum"=w406) -> (error out=w429:errorcluster)  [unwired: 1 in, 1 out]
        n210 = property on="Command" class="Bool (strict)"(error in=w429, "DisabledEnum"=w406) -> (error out=w428:errorcluster)  [unwired: 1 in, 1 out]
        n211 = property on="Go Home" class="Bool (strict)"(error in=w428, "DisabledEnum"=w406) -> (error out=w427:errorcluster)  [unwired: 1 in, 1 out]
        n212 = property on="Simulation" class="Bool (strict)"(error in=w427, "DisabledEnum"=w406) -> (error out=w418:errorcluster)  [unwired: 1 in, 1 out]
        n213 = while {
          tunnel: w418 -> [w463]
          tunnel: w419 -> [w458]
          tunnel: [w457] -> w426
          tunnel: [w463] -> w409
          tunnel: [w462] -> w415
          shift-right: [w461] -> _
          shift-left: w413 -> [w459]
          tunnel: w413 -> [w460]
          stop <- w462 stop-if-true
          n214 = event shown="[1] \"stop\": Value Change" {
            selector: _ -> [_ _ _]
            dyn-events: _ -> [_ _ _]
            timeout: w459 -> [_ _ _]
            tunnel: [w464 TRUE ("Finish Rotation") "Finish Rotation"] -> w462
            tunnel: [w475 _ w483] -> w461
            tunnel: w460 -> [w474 _ _]
            tunnel: w459 -> [_ _ w483]
            tunnel: w458 -> [w469 w480 w482]
            tunnel: [w468 w480 w482] -> w457
            tunnel: [w467 _ 0.0 ("Angle Time Step (ms)")] -> w456
            event Timeout; "Start/pause": Value Change {
              n215 = event-data() -> ()  [unwired: 1 in, 2 out]
              n216 = call "Simulation Angle Step (SubVI).vi"("n"="Polynomial Degree", "N (Rot)"="Number of Rotations", "Final Angle"="Final Angle (deg)", "VISA Refnum in"=w469) -> ("Next Angle"=w471:dbl, "VISA Refnum out"=w470:refnum<visa-resource-name>, "Angle Time Step (ms)"=w467:dbl, "Rotation Complete?"=w464:bool)  [unwired: 3 in, 1 out]
              n217 = case shown="True" "Start/pause" {
                tunnel: [w477 100] -> w475
                tunnel: w474 -> [w477 _]
                frame False {
                }
                frame True {
                }
              }
              n218 = call "Move Absolute (SubVI).vi"("Move to Angle"=w471, "VISA Refnum in"=w470) -> ("New Angle"=→"Current Angle":dbl, "VISA Refnum out"=w468:refnum<visa-resource-name>)  [unwired: 7 in, 1 out]
            }
            event "stop": Value Change {
              n219 = event-data() -> ()  [unwired: 1 in, 5 out]
            }
            event "Finish Rotation": Value Change {
              n220 = event-data() -> ()  [unwired: 1 in, 5 out]
            }
          }
          n221 = Wait (ms)(milliseconds to wait=w456) -> ()  [unwired: 1 out]
        }
        n222 = while {
          tunnel: w418 -> [w436]
          tunnel: w419 -> [w437]
          tunnel: [w437] -> _
          tunnel: [w436] -> w410
          shift-right: [w433] -> _
          shift-left: w412 -> [w434]
          tunnel: [w432] -> w414
          tunnel: w412 -> [w431]
          stop <- w432 stop-if-true
          # "SIMULATED STAGE MOVEMENT"
          n223 = event shown="[0] Timeout;  \"Start/Pause Stage\": Value Change" {
            selector: _ -> [_ _ _]
            dyn-events: _ -> [_ _ _]
            timeout: w434 -> [_ _ _]
            tunnel: [w447 TRUE ("Finish Stage") "Finish Stage"] -> w432
            tunnel: [w449 _ w454] -> w433
            tunnel: w434 -> [_ _ w454]
            tunnel: [w448 _ 0.0 ("Time Between Steps (ms)")] -> w435
            tunnel: w431 -> [w441 _ _]
            event Timeout; "Start/Pause Stage": Value Change {
              n224 = event-data() -> ()  [unwired: 1 in, 2 out]
              n225 = global write "Stage Global.vi" "Speed"("Speed (um/s)") -> ()
              n226 = global read "Stage Global.vi" "Position"() -> (w443:dbl)
              n227 = call "Slider Simulation Details (SubVI).vi"("Number of Steps"="Number of Steps") -> ("Time Between Steps (ms)"=w448:dbl, "Step Size (mm)"=w439:dbl)  [unwired: 9 in]
              n228 = global write "Stage Global.vi" "Final Position"("Final Position (mm)") -> ()
              n229 = Add(x=w443, y=w439) -> (x+y=w438:dbl)
              "Current Position (mm)" <- w438
              n230 = global read "Stage Global.vi" "Final Position"() -> (w440:dbl)
              n231 = case shown="True" "Start/Pause Stage" {
                tunnel: [w450 100] -> w449
                tunnel: w441 -> [w450 _]
                frame False {
                }
                frame True {
                }
              }
              n232 = global write "Stage Global.vi" "Position"(w438) -> ()
              n233 = Less Or Equal?(x=w440, y=w438) -> (x <= y?=w447:bool)
            }
            event "stop": Value Change {
              n234 = event-data() -> ()  [unwired: 1 in, 5 out]
            }
            event "Finish Stage": Value Change {
              n235 = event-data() -> ()  [unwired: 1 in, 1 out]
            }
          }
          n236 = Wait (ms)(milliseconds to wait=w435) -> ()  [unwired: 1 out]
        }
        n237 = And(x=w415, y=w414) -> (x .and. y?=w416:bool)
        n238 = Not(x=w416) -> (.not. x?=w408:bool)
        n239 = local write "Finish Rotation"(w408) -> ()
        n240 = local write "Finish Stage"(w408) -> ()
        n241 = local write "Simulate?"(w408) -> ()
        n242 = Select(t=w409, s=TRUE, f=w410) -> (s? t:f=w401:errorcluster)
        n243 = property on="Activate AngleScan" class="Bool (strict)"(error in=w401, "DisabledEnum"=w403) -> (error out=w402:errorcluster)  [unwired: 1 in, 1 out]
        n244 = property on="Simulation" class="Bool (strict)"(error in=w402, "DisabledEnum"=w403) -> (error out=w422:errorcluster)  [unwired: 1 in, 1 out]
        n245 = property on="Scan" class="Bool (strict)"(error in=w422, "DisabledEnum"=w403) -> (error out=w425:errorcluster)  [unwired: 1 in, 1 out]
        n246 = property on="Go Home" class="Bool (strict)"(error in=w425, "DisabledEnum"=w403) -> (error out=w424:errorcluster)  [unwired: 1 in, 1 out]
        n247 = property on="Command" class="Bool (strict)"(error in=w424, "DisabledEnum"=w403) -> (error out=w423:errorcluster)  [unwired: 1 in, 1 out]
        n248 = local read "stop"() -> (w430:bool)
        "Simulate?" <- "Simulation"
      }
      event "stop": Value Change {
        n249 = event-data() -> ()  [unwired: 1 in, 5 out]
        n250 = local read "stop"() -> (w487:bool)
      }
    }
    n251 = local write "stop"("stop") -> ()
    n252 = Or(x="stop", y=w26) -> (x .or. y?=w27:bool)
  }
  n253 = while {
    stop <- FALSE stop-if-true
    n254 = event shown="[2] \"Restore\": Value Change" {
      selector: _ -> [_ _ _]
      dyn-events: _ -> [_ _ _]
      timeout: _ -> [_ _ _]
      event Timeout {
        n255 = event-data() -> ()  [unwired: 1 in, 2 out]
      }
      event "Calibrate": Value Change {
        n256 = event-data() -> ()  [unwired: 1 in, 5 out]
        n257 = stacked-sequence {
          frame #0 {
            n258 = global read "GlobalUI.vi" "Stage Acquire Parameters"() -> (w499:T6)
            n259 = Unbundle By Name(w499) -> ("Start position mm"=w498:dbl, "End position mm"=w497:dbl)
            n260 = formula code="float64 m,b;\nm = 45/(xf-xi);\nb = -m*xi;"("xf"=w497, "xi"=w498) -> ("m"=w495:dbl, "b"=w496:dbl)
            n261 = Format Into String(w496) -> (resulting string=w493:string)  [unwired: 3 in, 1 out]
            n262 = Format Into String(w495) -> (resulting string=w494:string)  [unwired: 3 in, 1 out]
            n263 = local read "Rotation f(x) (mm -> deg)"() -> (w490:string)
            n264 = Concatenate Strings(w494, "*x + " ("string"), w493) -> (w489:string)
            n265 = Not Equal?(x=w490, y=w489) -> (x != y?=w491:bool)
            n266 = case shown="False" w491 {
              tunnel: w490 -> [_ w501]
              tunnel: w489 -> [_ w500]
              frame False {
              }
              frame True {
                n267 = stacked-sequence {
                  tunnel: w501 -> [w502 _]
                  tunnel: w500 -> [_ w503]
                  frame #0 {
                    n268 = local write "OriginalFormula"(w502) -> ()
                  }
                  frame #1 {
                    n269 = local write "Rotation f(x) (mm -> deg)"(w503) -> ()
                  }
                }
              }
            }
          }
        }
      }
      event "Restore": Value Change {
        n270 = event-data() -> ()  [unwired: 1 in, 5 out]
        n271 = local write "Rotation f(x) (mm -> deg)"("OriginalFormula") -> ()
      }
    }
  }
  n272 = call <instrlib>:"Close.vi"("error in (no error)"=w17, "VISA resource name"=w19) -> ("error out"=w16:errorcluster)  [unwired: 8 in, 1 out]
  n273 = call <vilib>:"General Error Handler.vi"("error in (no error)"=w16) -> ()  [unwired: 10 in, 5 out]
  "Calibrate?" <- w10
